vi "Deadband.vi"(11 "joystickValueIn":dbl) -> (3 "joystickValueOut":dbl)   [LabVIEW 2011]
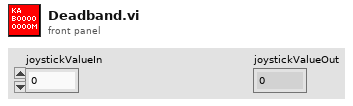
[diagram p1: front panel]
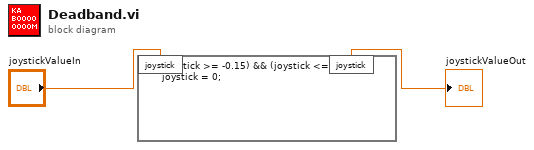
[diagram p0: block diagram]
diagram:
  n1 = formula code="if ((joystick >= -0.15) && (joystick <= 0.15))\n     joystick = 0;"("joystick"="joystickValueIn") -> ("joystick"=→"joystickValueOut":dbl)
